vi "Subtract Traces.vi"(5 "trace 2":string="Trace2" caption="trace 2 (Trace2)", 7 "trace 1":string="Trace1" caption="trace 1 (Trace1)", 8 "error in (no error)":errorcluster {"code" format="%.0x"}, 10 "destination trace":string="Trace3" caption="destination trace (Trace3)", 11 "instrument handle":refnum<k15>) -> (0 "error out":errorcluster {"code" format="%.0x"}, 3 "instrument handle out":refnum<k15>)   [LabVIEW 2009, in "Keysight XSAn.lvlib"]
doc: "This function subtracts the array elements of Trace 2 from Trace 1 and stores the result in the Destination Trace.\n\nSupported Models: All supported"
uses:
  <instrlib>/Keysight XSAn/Keysight XSAn.lvlib
  AgXSAn.dll
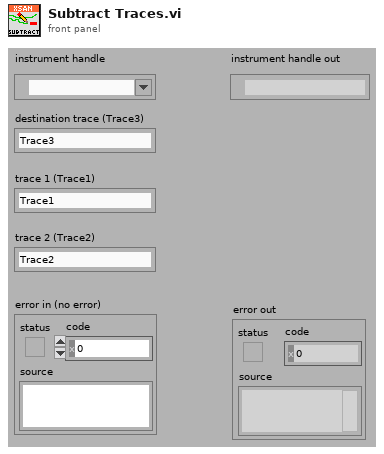
[diagram p1: front panel]
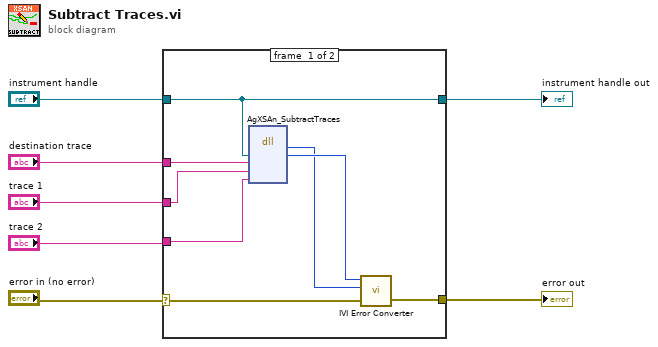
[diagram p0: block diagram]
diagram:
  n1 = case shown="No Error" "error in (no error)" {
    selector: "error in (no error)" -> [w13 w17]
    tunnel: [w14 w17] -> w6
    tunnel: "instrument handle" -> [w11 w16]
    tunnel: [w11 w16] -> w4
    tunnel: "trace 2" -> [w10 _]
    tunnel: "trace 1" -> [w9 _]
    tunnel: "destination trace" -> [w8 _]
    frame #0 {
      n2 = dll-call lib="AgXSAn**.dll" fn="AgXSAn_SubtractTraces" ("LabVIEW:IviSpecAn_SubtractTraces")("instrument handle"=w11, "destination trace"=w8, "trace 1"=w9, "trace 2"=w10) -> ("Status"=w12:i32, "instrument handle"=w15:u32)  [unwired: 6 in, 2 out]
      n3 = call <instrlib>:"IVI Error Converter.vi"("error in (no error)"=w13, "IVI error code (0)"=w12, "instrument handle"=w15) -> ("error out"=w14:errorcluster)  [unwired: 7 in, 1 out]
    }
    frame #1 {
    }
  }
  "error out" <- w6
  "instrument handle out" <- w4
